vi "ParseCmdArgs.vi"(10 "key":string, 11 "CmdArgs":string[](array[string])) -> (1 "found":bool, 2 "value":string)   [LabVIEW 2017]
panel:
  out "CmdArgs out":string[](array[string])
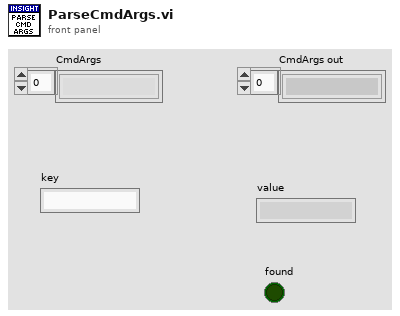
[diagram p1: front panel]
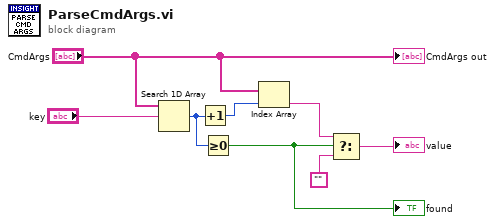
[diagram p0: block diagram]
diagram:
  n1 = Search 1D Array(1D array="CmdArgs", element="key") -> (index of element=w5:i32)  [unwired: 1 in]
  n2 = Increment(x=w5) -> (x+1=w6:i32)
  n3 = Greater Or Equal To 0?(x=w5) -> (x >= 0?=w4:bool)
  "found" <- w4
  n4 = Index Array(array="CmdArgs", index=w6) -> (element=w2:string)
  n5 = Select(t=w2, s=w4, f="") -> (s? t:f=→"value":string)
  "CmdArgs out" <- "CmdArgs"
